vi "PhotonPoseEstimator_closestToReferencePoseStrategy.vi"(9 "ReferencePose":T2={"Translation3d"={"X"=0.0, "Y"=0.0, "Z"=0.0}, "Rotation3d"={"Q_quaternion"={"R"=1.0, "V"=[0.0, 0.0, 0.0]}}} {"Translation3d"."Z" format="%14.3f"; "Translation3d"."Y" format="%14.3f"; "Translation3d"."X" format="%14.3f"}, 10 "CameraResult":T12 {"Targets"."AltCameraToTarget"."TRANSLATION3D"."Z" format="%14.3f"; "Targets"."AltCameraToTarget"."TRANSLATION3D"."Y" format="%14.3f"; "Targets"."AltCameraToTarget"."TRANSLATION3D"."X" format="%14.3f"; "Targets"."BestCameraToTarget"."TRANSLATION3D"."Z" format="%14.3f"; "Targets"."BestCameraToTarget"."TRANSLATION3D"."Y" format="%14.3f"; "Targets"."BestCameraToTarget"."TRANSLATION3D"."X" format="%14.3f"}, 11 "PhotoPoseEstimator":T1={"LastPose"={"Translation3d"={"X"=0.0, "Y"=0.0, "Z"=0.0}, "Rotation3d"={"Q_quaternion"={"R"=1.0, "V"=[0.0, 0.0, 0.0]}}}, "ReferencePose"={"Translation3d"={"X"=0.0, "Y"=0.0, "Z"=0.0}, "Rotation3d"={"Q_quaternion"={"R"=1.0, "V"=[0.0, 0.0, 0.0]}}}, "FieldTags"={"AprilTagMap"={}, "FieldLength"=0.0, "FieldWidth"=0.0, "OriginPosition "=enum."kBlueAllianceWallRightSide,", "OriginPose3d"={"Translation3d"={"X"=0.0, "Y"=0.0, "Z"=0.0}, "Rotation3d"={"Q_quaternion"={"R"=1.0, "V"=[0.0, 0.0, 0.0]}}}}, "PhotonPoseStrategy"=enum."LOWEST_AMBIGUITY", "Camera"="", "RobotToCamera"={"TRANSLATION3D"={"X"=0.0, "Y"=0.0, "Z"=0.0}, "ROTATION3D"={"Q_quaternion"={"R"=1.0, "V"=[0.0, 0.0, 0.0]}}, "XF"=FALSE}, "ReportedErrors"=[], "HighestAmbiguity"=10.0} {"RobotToCamera"."TRANSLATION3D"."Z" format="%14.3f"; "RobotToCamera"."TRANSLATION3D"."Y" format="%14.3f"; "RobotToCamera"."TRANSLATION3D"."X" format="%14.3f"; "FieldTags"."OriginPose3d"."Translation3d"."Z" format="%14.3f"; "FieldTags"."OriginPose3d"."Translation3d"."Y" format="%14.3f"; "FieldTags"."OriginPose3d"."Translation3d"."X" format="%14.3f"; "ReferencePose"."Translation3d"."Z" format="%14.3f"; "ReferencePose"."Translation3d"."Y" format="%14.3f"; "ReferencePose"."Translation3d"."X" format="%14.3f"; "LastPose"."Translation3d"."Z" format="%14.3f"; "LastPose"."Translation3d"."Y" format="%14.3f"; "LastPose"."Translation3d"."X" format="%14.3f"}) -> (1 "Pos Found":bool, 3 "PhotonEstimatedRobotPose":T11={"EstimatedPose"={"Translation3d"={"X"=0.0, "Y"=0.0, "Z"=0.0}, "Rotation3d"={"Q_quaternion"={"R"=1.0, "V"=[0.0, 0.0, 0.0]}}}, "TimeStamp_Seconds"=0.0} {"EstimatedPose"."Translation3d"."Z" format="%14.3f"; "EstimatedPose"."Translation3d"."Y" format="%14.3f"; "EstimatedPose"."Translation3d"."X" format="%14.3f"})   [LabVIEW 2019, in "PhotonVisionLib.lvlib"]
doc: "This is an internal function. Use Update or Update_Pipeline instead of this function.\n\nDetermine the best target based on the closest to a set Reference position"
uses:
  PhotonVisionLib.lvlib
  TypeDef/PhotonPipelineResultType.ctl
  TypeDef/PhotonTrackedTargetType.ctl
  TypeDef/TargetCornerType.ctl
  <vilib>/Rock Robotics/WPI/ThirdParty/JAS_Junk/TrajLib/TypeDef/TRANSFORM3D.ctl
  <vilib>/Rock Robotics/WPI/ThirdParty/JAS_Junk/TrajLib/TypeDef/TRANSLATION3D.ctl
  <vilib>/Rock Robotics/WPI/ThirdParty/JAS_Junk/TrajLib/TypeDef/ROTATION3D.ctl
  <vilib>/Rock Robotics/WPI/ThirdParty/JAS_Junk/TrajLib/TypeDef/QUATERNION.ctl
  TypeDef/PhotonEstimatedRobotPoseType.ctl
  <vilib>/Rock Robotics/WPI/ThirdParty/JAS_Junk/TrajLib/TypeDef/POSE3D.ctl
  TypeDef/PhotonPoseEstimatorType.ctl
  <vilib>/Rock Robotics/WPI/ThirdParty/JAS_Junk/TrajLib/TypeDef/AprilTagFieldLayout.ctl
  <vilib>/Rock Robotics/WPI/ThirdParty/JAS_Junk/TrajLib/TypeDef/AprilTag.ctl
  <vilib>/Rock Robotics/WPI/ThirdParty/JAS_Junk/TrajLib/Enum/AprilTagFieldLayoutOrignPosition_ENUM.ctl
  TypeDef/PhotonPoseStrategy_ENUM.ctl
  <vilib>/Rock Robotics/WPI/ThirdParty/JAS_Junk/TrajLib/VI/AprilTag_GetAll.vi
  <vilib>/Rock Robotics/WPI/ThirdParty/JAS_Junk/TrajLib/VI/Pose3d_RelativeTo.vi
  <vilib>/Rock Robotics/WPI/ThirdParty/JAS_Junk/TrajLib/VI/Transform3d_GetRotation3d.vi
  <vilib>/Rock Robotics/WPI/ThirdParty/JAS_Junk/TrajLib/VI/Transform3d_GetTranslation3d.vi
  <vilib>/Rock Robotics/WPI/ThirdParty/JAS_Junk/TrajLib/VI/Translation3d_ToTranslation2d.vi
  <vilib>/Rock Robotics/WPI/ThirdParty/JAS_Junk/TrajLib/VI/Rotation3d_ToRotation2d.vi
  <vilib>/Rock Robotics/WPI/ThirdParty/JAS_Junk/TrajLib/Transform2d_Create_TransRot.vi
  <vilib>/Rock Robotics/WPI/ThirdParty/JAS_Junk/TrajLib/VI/Pose3d_TransformBy.vi
  <vilib>/Rock Robotics/WPI/ThirdParty/JAS_Junk/TrajLib/VI/Transform3d_Inverse.vi
  PhotonPoseEstimator_CalcDifference.vi
  <vilib>/Rock Robotics/WPI/ThirdParty/JAS_Junk/TrajLib/VI/Rotation3d_Create_AxisAngle.vi
  <vilib>/Rock Robotics/WPI/ThirdParty/JAS_Junk/TrajLib/VI/Pose3d_New.vi
  <vilib>/Rock Robotics/WPI/ThirdParty/JAS_Junk/TrajLib/VI/Pose3d_New_Trans3dRot3d.vi
  <vilib>/Rock Robotics/WPI/ThirdParty/JAS_Junk/TrajLib/VI/Transform3d_Create_Pose3dPose3d.vi
  <vilib>/Rock Robotics/WPI/ThirdParty/JAS_Junk/TrajLib/Translation2d_Create.vi
  <vilib>/Rock Robotics/WPI/ThirdParty/JAS_Junk/TrajLib/Rotation2d_CreateAngle.vi
  <vilib>/Rock Robotics/WPI/ThirdParty/JAS_Junk/TrajLib/VI/Rotation3d_GetXYZ.vi
  <vilib>/Rock Robotics/WPI/ThirdParty/JAS_Junk/TrajLib/VI/Pose3d_getTranslation3d.vi
  <vilib>/Rock Robotics/WPI/ThirdParty/JAS_Junk/TrajLib/VI/Pose3d_getRotation3d.vi
  <vilib>/Rock Robotics/WPI/ThirdParty/JAS_Junk/TrajLib/VI/Translation3d_Plus.vi
  <vilib>/Rock Robotics/WPI/ThirdParty/JAS_Junk/TrajLib/VI/Translation3d_RotateBy.vi
  <vilib>/Rock Robotics/WPI/ThirdParty/JAS_Junk/TrajLib/VI/Rotation3d_Plus.vi
  <vilib>/Rock Robotics/WPI/ThirdParty/JAS_Junk/TrajLib/VI/Transform3d_Create_Trans3dRot3d.vi
  <vilib>/Rock Robotics/WPI/ThirdParty/JAS_Junk/TrajLib/VI/Rotation3d_UnaryMinus.vi
  <vilib>/Rock Robotics/WPI/ThirdParty/JAS_Junk/TrajLib/VI/Translation3d_UnaryMinus.vi
  <vilib>/Rock Robotics/WPI/ThirdParty/JAS_Junk/TrajLib/VI/Translation3d_GetDistance.vi
  <vilib>/Rock Robotics/WPI/ThirdParty/JAS_Junk/TrajLib/VI/Quaternion_New.vi
  <vilib>/Rock Robotics/WPI/ThirdParty/JAS_Junk/TrajLib/VI/Rotation3d_Create_Default.vi
  <vilib>/Rock Robotics/WPI/ThirdParty/JAS_Junk/TrajLib/VI/Vector_Norm.vi
  <vilib>/Rock Robotics/WPI/ThirdParty/JAS_Junk/TrajLib/VecBuilder_ArrayBy1Fill.vi
  <vilib>/Rock Robotics/WPI/ThirdParty/JAS_Junk/TrajLib/VI/Translation3d_Create.vi
  <vilib>/Rock Robotics/WPI/ThirdParty/JAS_Junk/TrajLib/VI/Translation3d_Minus.vi
  <vilib>/Rock Robotics/WPI/ThirdParty/JAS_Junk/TrajLib/VI/Rotation3d_Minus.vi
  <vilib>/Rock Robotics/WPI/ThirdParty/JAS_Junk/TrajLib/VI/Quaternion_Get_All.vi
  <vilib>/Rock Robotics/WPI/ThirdParty/JAS_Junk/TrajLib/VI/Rotation3d_GetQuaterion.vi
  <vilib>/Rock Robotics/WPI/ThirdParty/JAS_Junk/TrajLib/VI/Quaternion_Times.vi
  <vilib>/Rock Robotics/WPI/ThirdParty/JAS_Junk/TrajLib/VI/Quaternion_Inverse.vi
  <vilib>/Rock Robotics/WPI/ThirdParty/JAS_Junk/TrajLib/VI/Rotation3d_RotateBy.vi
  <vilib>/Rock Robotics/WPI/ThirdParty/JAS_Junk/TrajLib/VI/Rotation3d_Create_Quaternion.vi
  <vilib>/Rock Robotics/WPI/ThirdParty/JAS_Junk/TrajLib/VI/Quaternion_New_Default.vi
  <vilib>/Rock Robotics/WPI/ThirdParty/JAS_Junk/TrajLib/MatBuilder_Create.vi
  <vilib>/Rock Robotics/WPI/ThirdParty/JAS_Junk/TrajLib/VI/Quaternion_Normalize.vi
  <vilib>/Rock Robotics/WPI/ThirdParty/JAS_Junk/TrajLib/Trajectory_Library.lvlib
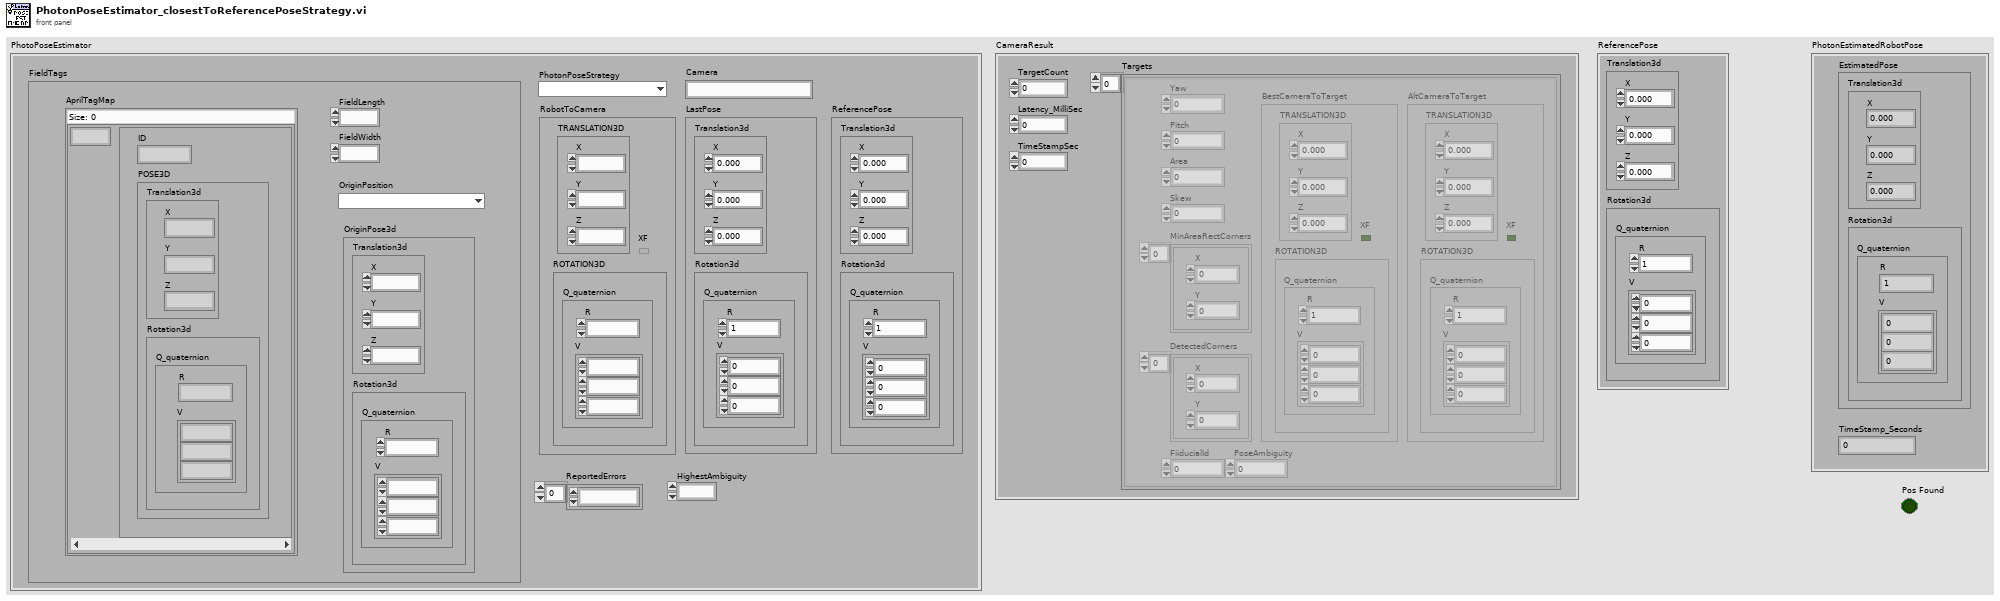
[diagram p1: front panel]
types:
  T1 = typedef "PhotonVisionLib.lvlib/PhotonPoseEstimatorType.ctl" = cluster{"LastPose":T2, "ReferencePose":T2, "FieldTags":T6, "PhotonPoseStrategy":T9, "Camera":string, "RobotToCamera":T10, "ReportedErrors":dbl[], "HighestAmbiguity":dbl}
  T2 = typedef "Trajectory_Library.lvlib/POSE3D.ctl" = cluster{"Translation3d":T3, "Rotation3d":T4}
  T3 = typedef "Trajectory_Library.lvlib/TRANSLATION3D.ctl" = cluster{"X":dbl, "Y":dbl, "Z":dbl}
  T4 = typedef "Trajectory_Library.lvlib/ROTATION3D.ctl" = cluster{"Q_quaternion":T5}
  T5 = typedef "Trajectory_Library.lvlib/QUATERNION.ctl" = cluster{"R":dbl, "V":dbl[]}
  T6 = typedef "Trajectory_Library.lvlib/AprilTagFieldLayout.ctl" = cluster{"AprilTagMap":map{i32, T7}, "FieldLength":dbl, "FieldWidth":dbl, "OriginPosition ":T8, "OriginPose3d":T2}
  T7 = typedef "Trajectory_Library.lvlib/AprilTag.ctl" = cluster{"ID":i32, "POSE3D":T2}
  T8 = typedef "Trajectory_Library.lvlib/AprilTagFieldLayoutOrignPosition_ENUM.ctl" = enum16{"kBlueAllianceWallRightSide,", "kRedAllianceWallRightSide,"}
  T9 = typedef "PhotonVisionLib.lvlib/PhotonPoseStrategy_ENUM.ctl" = enum16{"LOWEST_AMBIGUITY", "CLOSEST_TO_CAMERA_HEIGHT", "CLOSEST_TO_REFERENCE_POSE", "CLOSEST_TO_LAST_POSE", "AVERAGE_BEST_TARGETS"}
  T10 = typedef "Trajectory_Library.lvlib/TRANSFORM3D.ctl" = cluster{"TRANSLATION3D":T3, "ROTATION3D":T4, "XF":bool}
  T11 = typedef "PhotonVisionLib.lvlib/PhotonEstimatedRobotPoseType.ctl" = cluster{"EstimatedPose":T2, "TimeStamp_Seconds":dbl}
  T12 = typedef "PhotonVisionLib.lvlib/PhotonPipelineResultType.ctl" = cluster{"TargetCount":i32, "Latency_MilliSec":dbl, "Targets":T13[], "TimeStampSec":dbl}
  T13 = typedef "PhotonVisionLib.lvlib/PhotonTrackedTargetType.ctl" = cluster{"Yaw":dbl, "Pitch":dbl, "Area":dbl, "Skew":dbl, "MinAreaRectCorners":T14[], "BestCameraToTarget":T10, "FiiducialId":i32, "AltCameraToTarget":T10, "PoseAmbiguity":dbl, "DetectedCorners":T14[]}
  T14 = typedef "PhotonVisionLib.lvlib/TargetCornerType.ctl" = cluster{"X":dbl, "Y":dbl}
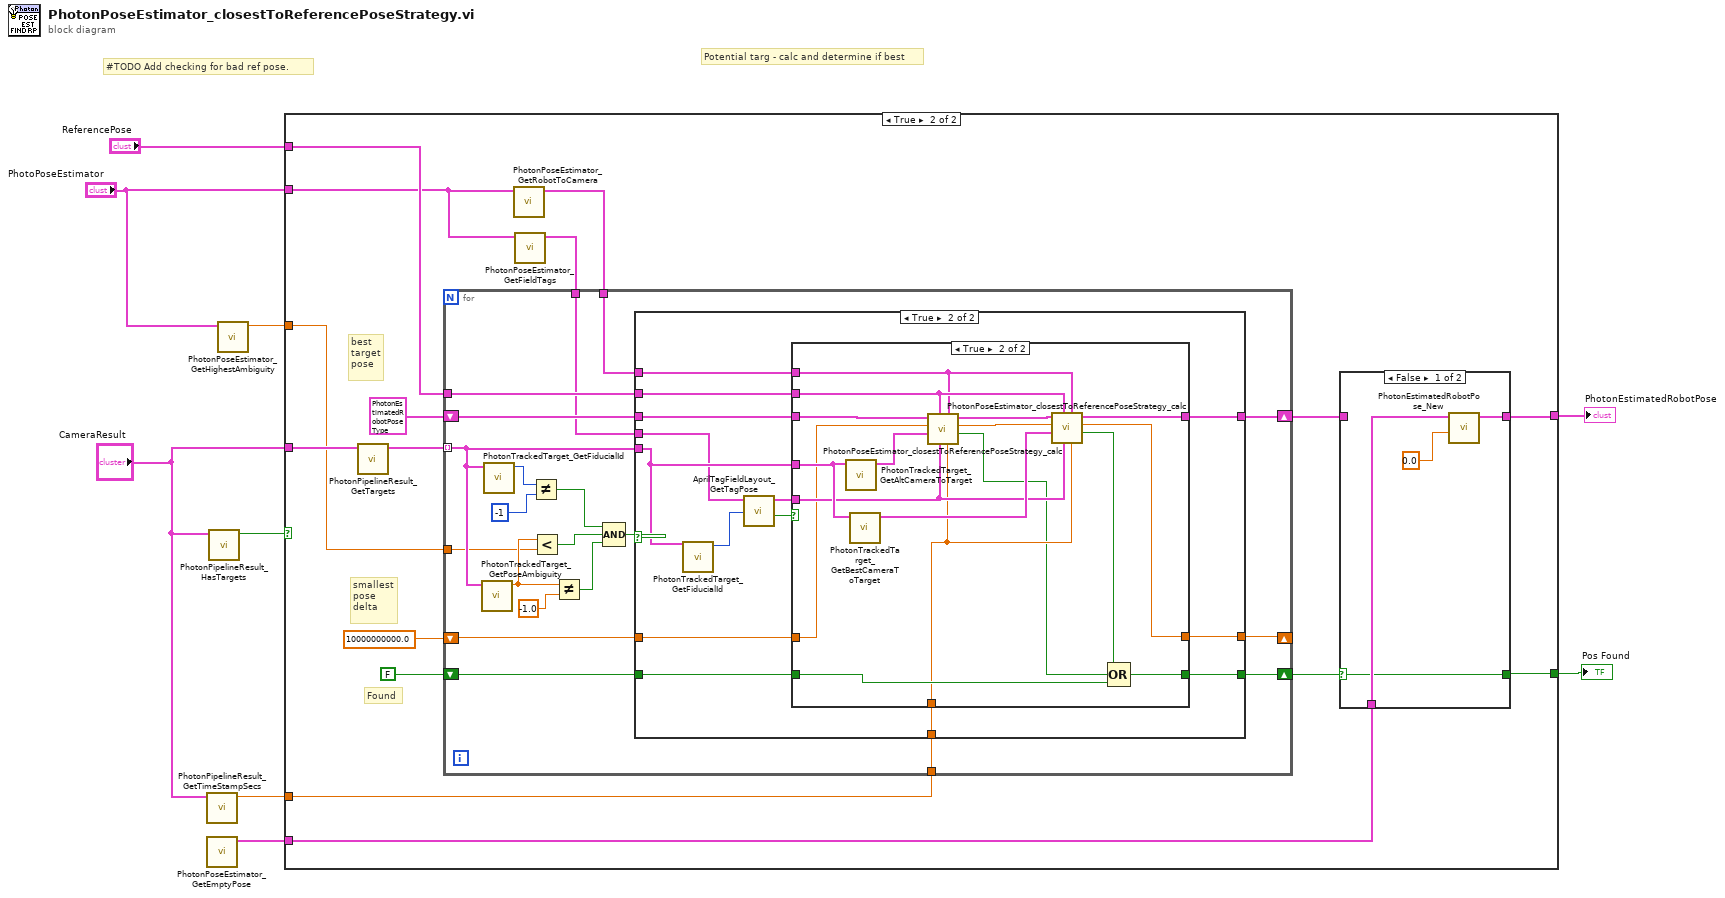
[diagram p0: block diagram]
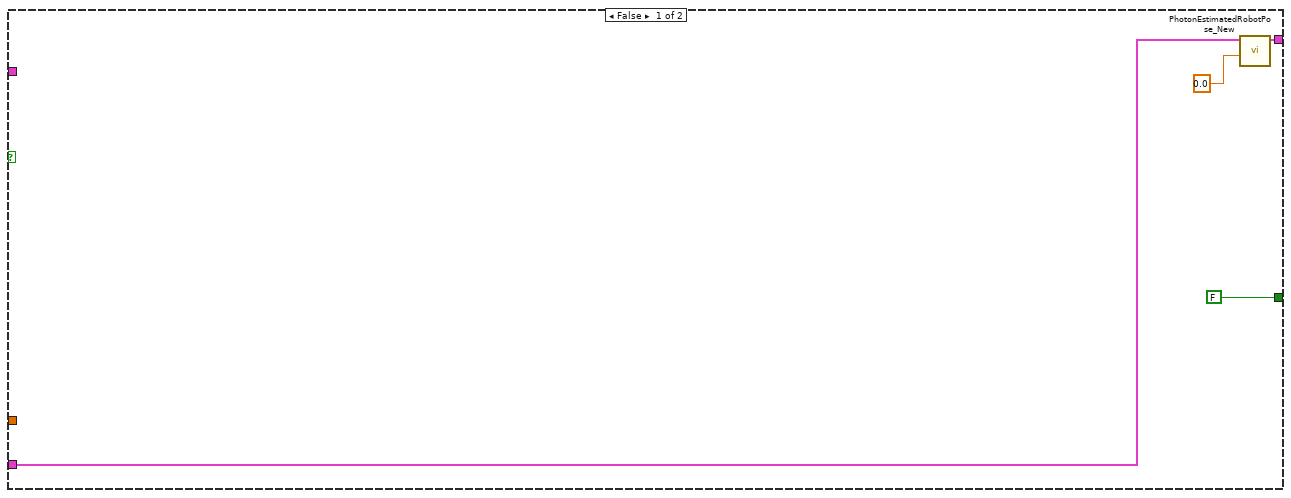
[diagram p2: hidden frame]
diagram:
  # "#TODO Add checking for bad ref pose."
  # "Potential targ - calc and determine if best"
  n1 = call "PhotonPipelineResult_GetTimeStampSecs.vi"("PhotonPipelineResult"="CameraResult") -> ("TimeStampSec"=w8:dbl)  [unwired: 10 in]
  n2 = call "PhotonPoseEstimator_GetEmptyPose.vi"() -> ("EmptyPose"=w7:T2)  [unwired: 11 in]
  n3 = call "PhotonPipelineResult_HasTargets.vi"("PhotonPipelineResult"="CameraResult") -> ("HasTargets"=w9:bool)  [unwired: 10 in]
  n4 = call "PhotonPoseEstimator_GetHighestAmbiguity.vi"("PhotonPoseEstimator"="PhotoPoseEstimator") -> ("HighestAmbiguity"=w1:dbl)  [unwired: 10 in]
  n5 = case shown="True" w9 {
    tunnel: "CameraResult" -> [_ w26]
    tunnel: [FALSE ("Found") w22] -> w3
    tunnel: "PhotoPoseEstimator" -> [_ w15]
    tunnel: w8 -> [_ w24]
    tunnel: [w11 w20] -> w4
    tunnel: w7 -> [w10 w19]
    tunnel: "ReferencePose" -> [_ w17]
    tunnel: w1 -> [_ w18]
    frame False {
      n6 = call "PhotonEstimatedRobotPose_New.vi"("TimeStamp_Seconds"=0.0, "EstimatedPose"=w10) -> ("PhotonEstimatedRobotPose"=w11:T11)  [unwired: 9 in]
    }
    frame True {
      # "smallest\npose\ndelta"
      # "best \ntarget\npose"
      # "Found"
      n7 = call "PhotonPipelineResult_GetTargets.vi"("PhotonPipelineResult"=w26) -> ("Targets"=w29:T13[])  [unwired: 10 in]
      n8 = call "PhotonPoseEstimator_GetRobotToCamera.vi"("PhotonPoseEstimator"=w15) -> ("RobotToCamera"=w14:T10)  [unwired: 10 in]
      n9 = call "PhotonPoseEstimator_GetFieldTags.vi"("PhotonPoseEstimator"=w15) -> ("AprilTagFieldLayout"=w16:T6)  [unwired: 10 in]
      n10 = for {
        tunnel: w29 -> [w47] mode=indexing
        shift-right: [w51] -> w21
        shift-left: T11 {"EstimatedPose"={"Translation3d"={"X"=0.0, "Y"=0.0, "Z"=0.0}, "Rotation3d"={"Q_quaternion"={"R"=1.0, "V"=[0.0, 0.0, 0.0]}}}, "TimeStamp_Seconds"=0.0} ("PhotonEstimatedRobotPose") -> [w50]
        shift-right: [w55] -> w23
        shift-left: FALSE -> [w52]
        shift-right: [w54] -> _
        shift-left: 10000000000.0 -> [w53]
        tunnel: w24 -> [w43]
        tunnel: w18 -> [w39]
        tunnel: w17 -> [w38]
        tunnel: w16 -> [w37]
        tunnel: w14 -> [w36]
        n11 = call "PhotonTrackedTarget_GetPoseAmbiguity.vi"("TrackedTarget"=w47) -> ("Pose Ambiguity"=w42:dbl)  [unwired: 10 in]
        n12 = call "PhotonTrackedTarget_GetFiducialId.vi"("TrackedTarget"=w47) -> ("Fiducial Id"=w49:i32)  [unwired: 10 in]
        n13 = Not Equal?(x=w49, y=-1) -> (x != y?=w41:bool)
        n14 = Less?(x=w42, y=w39) -> (x < y?=w40:bool)
        n15 = Not Equal?(x=w42, y=-1.0) -> (x != y?=w45:bool)
        n16 = Compound Arithmetic op=AND(w41, w40, w45) -> (w44:bool)
        n17 = case shown="True" w44 {
          tunnel: [w57 w65] -> w55
          tunnel: [w58 w71] -> w54
          tunnel: w53 -> [w58 w64]
          tunnel: w52 -> [w57 w63]
          tunnel: w47 -> [_ w69]
          tunnel: [w56 w70] -> w51
          tunnel: w50 -> [w56 w72]
          tunnel: w43 -> [_ w62]
          tunnel: w38 -> [_ w61]
          tunnel: w37 -> [_ w60]
          tunnel: w36 -> [_ w59]
          frame False {
          }
          frame True {
            n18 = call "PhotonTrackedTarget_GetFiducialId.vi"("TrackedTarget"=w69) -> ("Fiducial Id"=w68:i32)  [unwired: 10 in]
            n19 = call <vilib>:"AprilTagFieldLayout_GetTagPose.vi"("TagId"=w68, "AprilTagFieldLayout"=w60) -> ("Found"=w67:bool, "TagPose3d"=w66:T2)  [unwired: 8 in]
            n20 = case shown="True" w67 {
              tunnel: w72 -> [w75 w79]
              tunnel: [w74 w90] -> w71
              tunnel: [w75 w89] -> w70
              tunnel: w69 -> [_ w88]
              tunnel: w66 -> [_ w87]
              tunnel: [w73 w86] -> w65
              tunnel: w64 -> [w74 w78]
              tunnel: w63 -> [w73 w85]
              tunnel: w62 -> [_ w84]
              tunnel: w61 -> [_ w77]
              tunnel: w59 -> [_ w76]
              frame False {
              }
              frame True {
                n21 = call "PhotonTrackedTarget_GetAltCameraToTarget.vi"("TrackedTarget"=w88) -> ("AltCameraToTarget"=w91:T10)  [unwired: 9 in, 1 out]
                n22 = call "PhotonTrackedTarget_GetBestCameraToTarget.vi"("TrackedTarget"=w88) -> ("BestCameraToTarget"=w92:T10)  [unwired: 9 in, 1 out]
                n23 = call "PhotonPoseEstimator_closestToReferencePoseStrategy_calc.vi"("TimeStamp"=w84, "RobotToCamera"=w76, "FieldTargetPose"=w87, "Reference Pose"=w77, "TransformToEvaluate"=w91, "SmallestDistToReff"=w78, "CurrentBestTrackedTarg"=w79) -> ("Found New Best"=w82:bool, "SmallestDistToRef"=w81:dbl, "PhotonEstimatedRobotPose"=w80:T11)  [unwired: 2 in]
                n24 = call "PhotonPoseEstimator_closestToReferencePoseStrategy_calc.vi"("TimeStamp"=w84, "RobotToCamera"=w76, "FieldTargetPose"=w87, "Reference Pose"=w77, "TransformToEvaluate"=w92, "SmallestDistToReff"=w81, "CurrentBestTrackedTarg"=w80) -> ("Found New Best"=w83:bool, "SmallestDistToRef"=w90:dbl, "PhotonEstimatedRobotPose"=w89:T11)  [unwired: 2 in]
                n25 = Compound Arithmetic op=OR(w83, w82, w85) -> (w86:bool)
              }
            }
          }
        }
      }
      n26 = case shown="False" w23 {
        selector: w23 -> [w30 w35]
        tunnel: [w30 w35] -> w22
        tunnel: [w31 w34] -> w20
        tunnel: w21 -> [_ w34]
        tunnel: w19 -> [w32 _]
        frame False {
          n27 = call "PhotonEstimatedRobotPose_New.vi"("TimeStamp_Seconds"=0.0, "EstimatedPose"=w32) -> ("PhotonEstimatedRobotPose"=w31:T11)  [unwired: 9 in]
        }
        frame True {
        }
      }
    }
  }
  "PhotonEstimatedRobotPose" <- w4
  "Pos Found" <- w3
